vi "Connection Mode Generation Get Next Messages.vi"(0 "Connection Cluster":T2 {"Packets"."Identifier" format="%08x"}, 11 "error in (no error)":errorcluster) -> (4 "Connection Cluster":T2 {"Packets"."Identifier" format="%08x"}, 6 "Data to Send Array":T1[](array[typedef]) {"Identifier" format="%08x"}, 8 "Timeout?":bool, 10 "Message Available?":bool, 15 "error out":errorcluster)   [LabVIEW 2013, in "J1939.lvlib"]
uses:
  J1939.lvlib
  Connection Mode Generation Connection Cluster.ctl
  API Types/CAN Outgoing Message Cluster.ctl
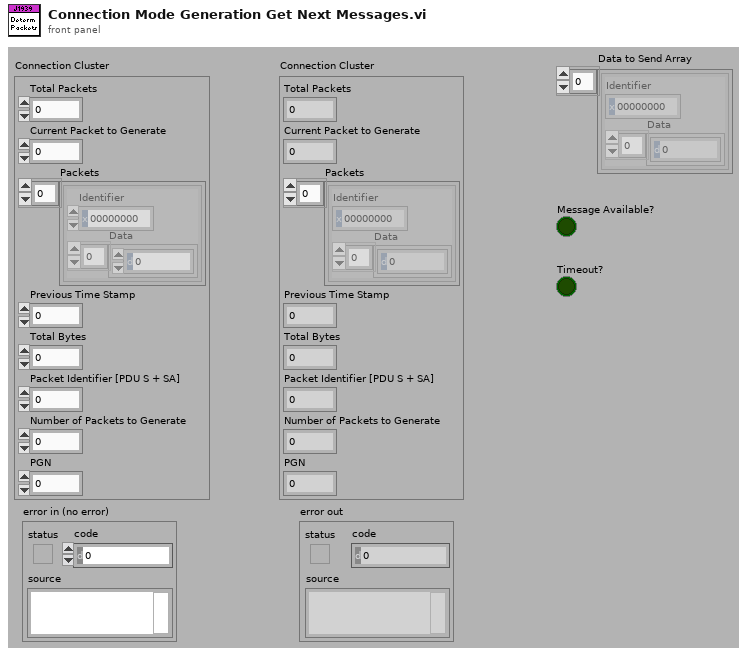
[diagram p1: front panel]
types:
  T1 = typedef "J1939.lvlib/CAN Outgoing Message Cluster.ctl" = cluster{"Identifier":u32, "Data":u8[]}
  T2 = typedef "J1939.lvlib/Connection Mode Generation Connection Cluster.ctl" = cluster{"Total Packets":u8, "Current Packet to Generate":u8, "Packets":T1[], "Previous Time Stamp":u32, "Total Bytes":u16, "Packet Identifier [PDU S + SA]":u16, "Number of Packets to Generate":u8, "PGN":u32}
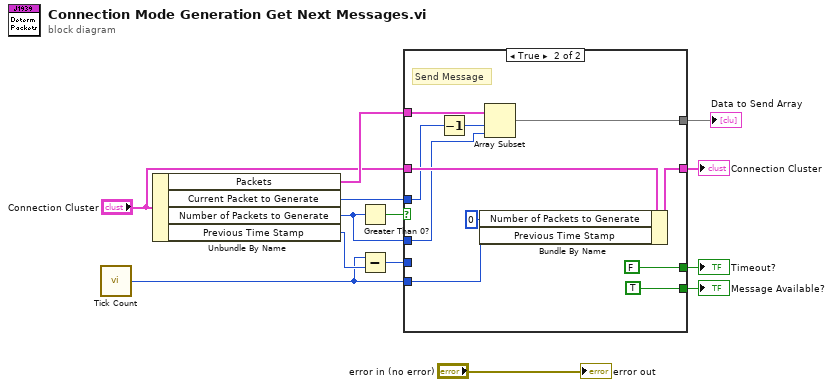
[diagram p0: block diagram]
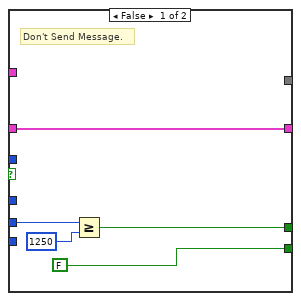
[diagram p2: hidden frame]
diagram:
  n1 = call "Tick Count"() -> ("Tick Count(mSec)"=w3:u32)
  n2 = Unbundle By Name("Connection Cluster") -> ("Packets"=w10:T1[], "Current Packet to Generate"=w9:u8, "Number of Packets to Generate"=w13:u8, "Previous Time Stamp"=w11:u32)
  n3 = Greater Than 0?(x=w13) -> (x > 0?=w2:bool)
  n4 = Subtract(x=w3, y=w11) -> (x-y=w12:u32)
  n5 = case shown="True" w2 {
    tunnel: w9 -> [_ w20]
    tunnel: [_ w23] -> w1
    tunnel: "Connection Cluster" -> [w18 w27]
    tunnel: [w18 w29] -> w7
    tunnel: w13 -> [_ w19]
    tunnel: w10 -> [_ w28]
    tunnel: w12 -> [w17 _]
    tunnel: [w16 FALSE] -> w6
    tunnel: w3 -> [_ w26]
    tunnel: [FALSE TRUE] -> w4
    frame False {
      # "Don't Send Message."
      n6 = Greater Or Equal?(x=w17, y=u32 1250) -> (x >= y?=w16:bool)
    }
    frame True {
      # "Send Message"
      n7 = Decrement(x=w20) -> (x-1=w22:u8)
      n8 = Bundle By Name(cluster=w27, "Number of Packets to Generate"=u8 0, "Previous Time Stamp"=w26) -> (w29:T2)
      n9 = Array Subset(array=w28, index=w22, length=w19) -> (w23:T1[])
    }
  }
  "Timeout?" <- w6
  "Connection Cluster" <- w7
  "Message Available?" <- w4
  "Data to Send Array" <- w1
  "error out" <- "error in (no error)"
